vi "project_file_read.vi"(8 "error in (no error)":errorcluster, 11 "lv-build in":refnum<class "lv-builder-l3.lvclass">) -> (0 "error out":errorcluster, 2 "project_file":path, 3 "lv-build out":refnum<class "lv-builder-l3.lvclass">)   [LabVIEW 2015, in "lv-builder-l3.lvlib" / "lv-builder-l3.lvclass"]
uses:
  lv-builder-l3.lvclass
  lv-builder/class/lv-builder.lvclass
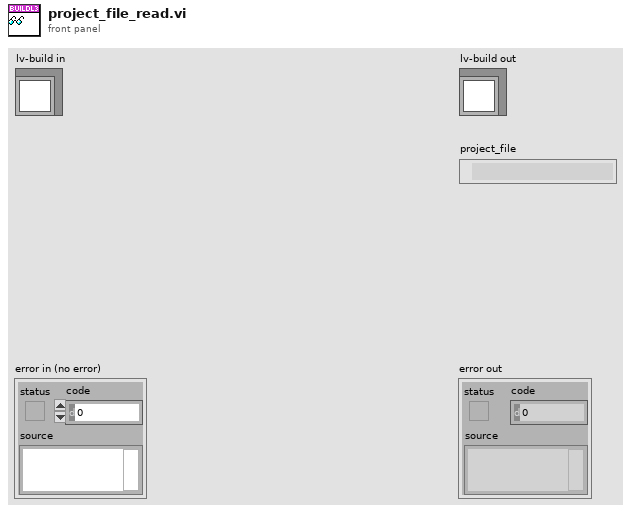
[diagram p1: front panel]
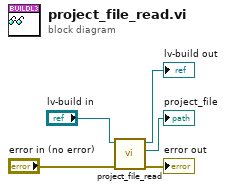
[diagram p0: block diagram]
diagram:
  n1 = call-parent "project_file_read.vi"("error in (no error)"="error in (no error)", "lv-build in"="lv-build in") -> ("error out"=→"error out":errorcluster, "project_file"=→"project_file":path, "lv-build out"=→"lv-build out":refnum<class "lv-builder-l3.lvclass">)  [unwired: 7 in]
